vi "Trajectories2 String.vi"(5 "Trajectories":T3[](array[typedef])) -> (2 "VPL":string)   [LabVIEW 2014]
uses:
  PBFAM/Controller/MachineController/Converters/ScanSub/Trajectory.ctl
  PBFAM/Controller/MachineController/Converters/ScanSub/Path.ctl
  PBFAM/Controller/MachineController/Converters/ScanSub/Point.ctl
  PBFAM/Controller/MachineController/Converters/ScanSub/Segment.ctl
panel:
  out "Start":T1
  out "End":cluster{"X":sgl, "Y":sgl}
  out "Array":string[](array[string])
  out "Segment":T2
  out "Path0":T4
  out "Trajectory":T3
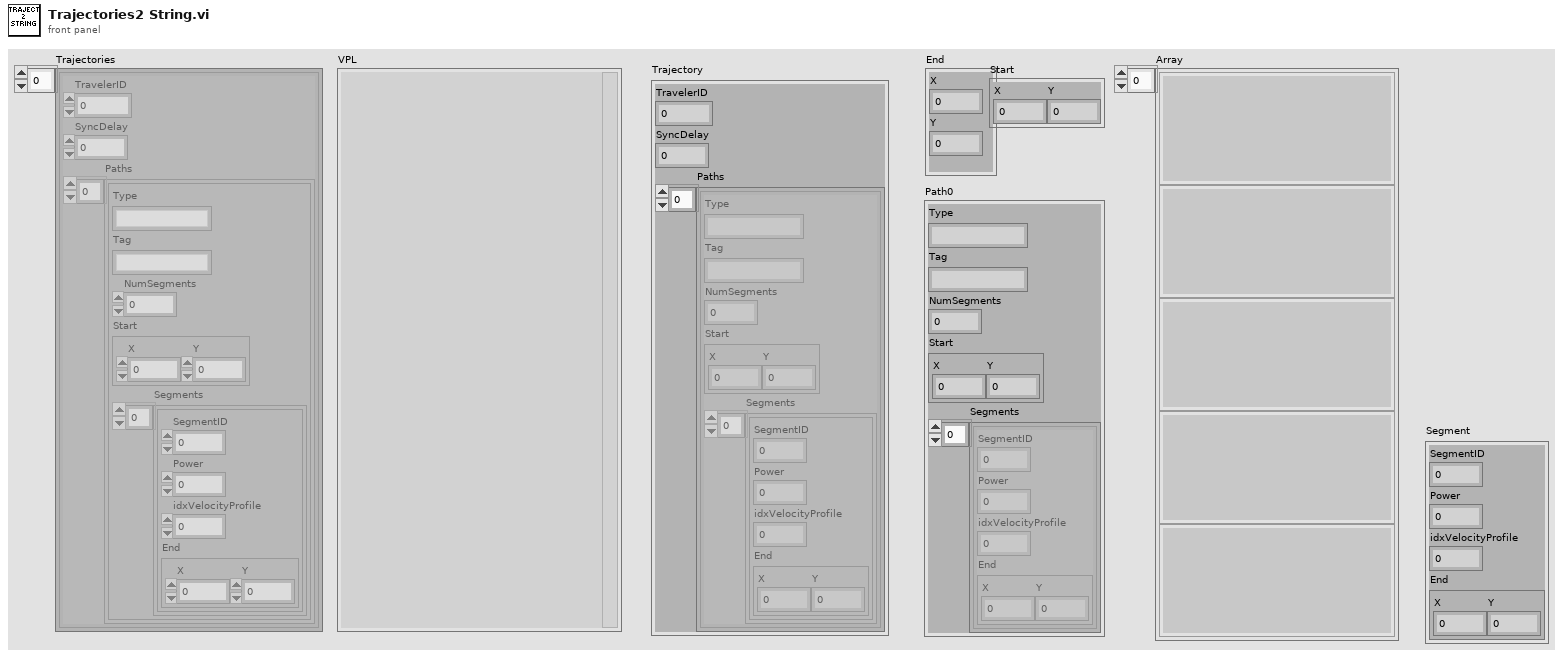
[diagram p1: front panel]
types:
  T1 = typedef "Point.ctl" = cluster{"X":dbl, "Y":dbl}
  T2 = typedef "Segment.ctl" = cluster{"SegmentID":u16, "Power":sgl, "idxVelocityProfile":u16, "End":cluster{"X":sgl, "Y":sgl}}
  T3 = typedef "Trajectory.ctl" = cluster{"TravelerID":u32, "SyncDelay":u32, "Paths":T4[]}
  T4 = typedef "Path.ctl" = cluster{"Type":string, "Tag":string, "NumSegments":u64, "Start":T1, "Segments":T2[]}
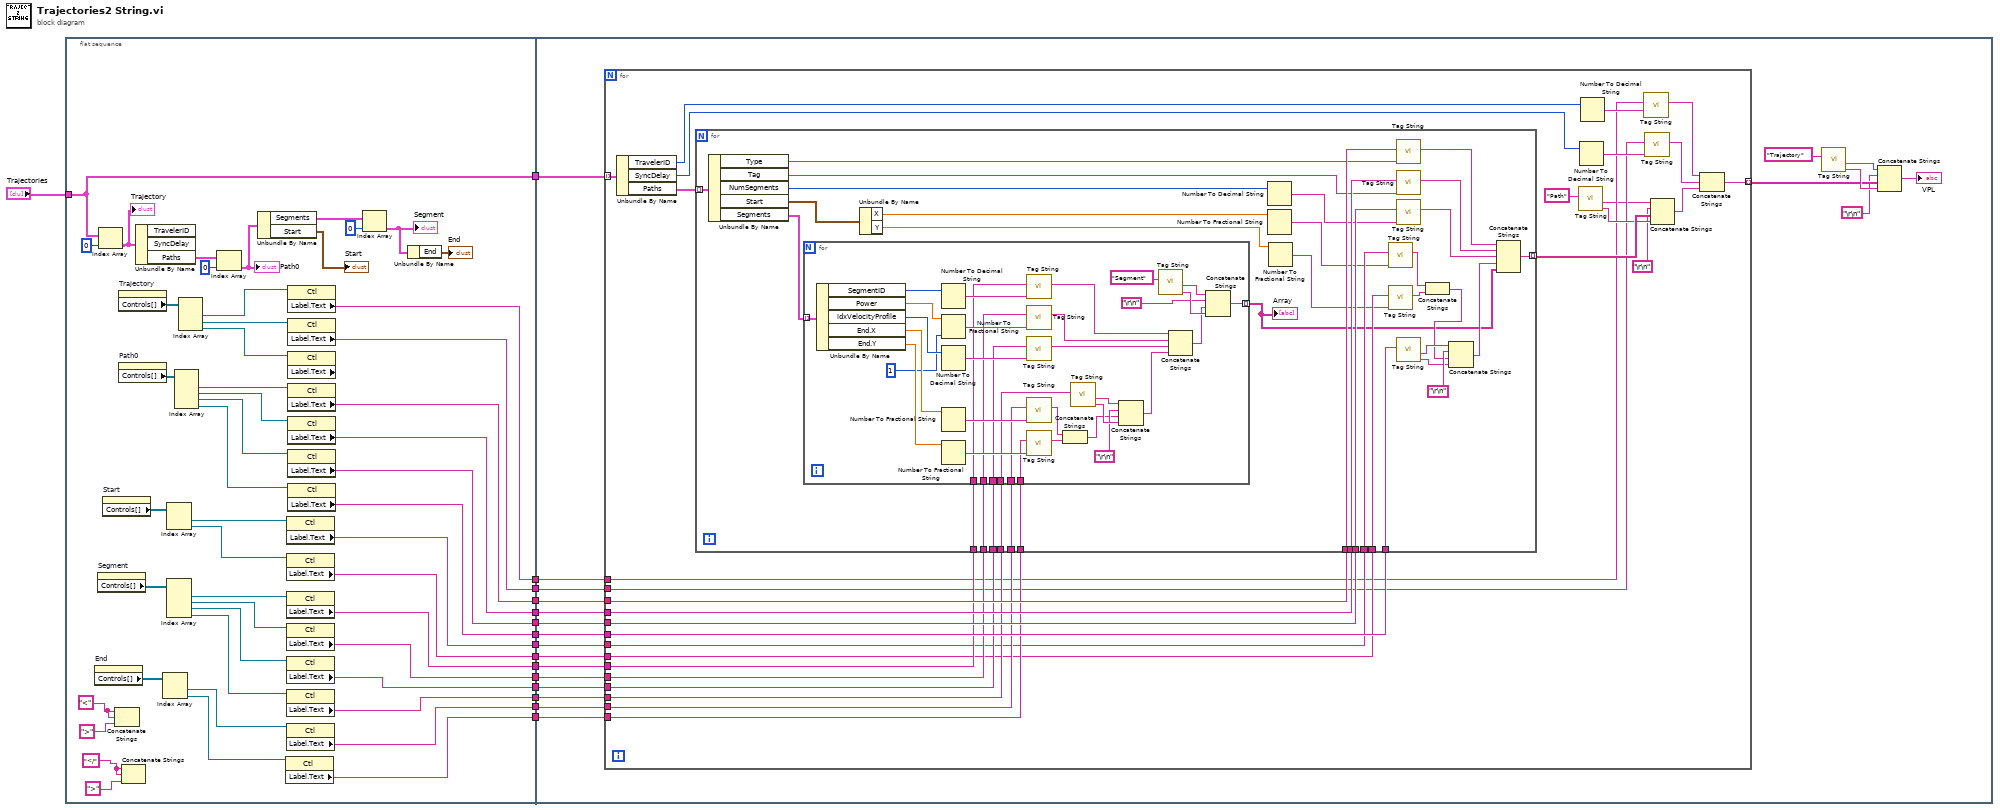
[diagram p0: block diagram]
diagram:
  n1 = flat-sequence {
    tunnel: [w53] -> w16
    tunnel: [w43] -> w15
    tunnel: [w42] -> w14
    tunnel: [w41] -> w13
    tunnel: [w40] -> w12
    tunnel: [w39] -> w11
    tunnel: [w38] -> w10
    tunnel: "Trajectories" -> [w53]
    tunnel: [w37] -> w8
    tunnel: [w36] -> w7
    tunnel: [w35] -> w6
    tunnel: [w34] -> w5
    tunnel: [w20] -> w4
    tunnel: [w19] -> w3
    tunnel: [w18] -> w2
    tunnel: [w17] -> w1
    tunnel: w16 -> [w86]
    tunnel: w15 -> [w85]
    tunnel: w14 -> [w84]
    tunnel: w13 -> [w83]
    tunnel: w12 -> [w82]
    tunnel: w11 -> [w81]
    tunnel: w10 -> [w80]
    tunnel: w8 -> [w79]
    tunnel: w7 -> [w78]
    tunnel: w6 -> [w77]
    tunnel: w5 -> [w76]
    tunnel: w4 -> [w75]
    tunnel: w3 -> [w74]
    tunnel: w2 -> [w73]
    tunnel: w1 -> [w72]
    frame #0 {
      w25 = "</" ("string")
      w26 = "<" ("string")
      n2 = property on="End" class="Clust (strict)"() -> ("Controls[]"=w31:refnum<vi>[])  [unwired: 2 in, 2 out]
      n3 = property on="Segment" class="Clust (strict)"() -> ("Controls[]"=w48:refnum<vi>[])  [unwired: 2 in, 2 out]
      n4 = Index Array(array=w53, index=0) -> (element=w52:T3)
      "Trajectory" <- w52
      n5 = property on="Start" class="Clust (strict)"() -> ("Controls[]"=w23:refnum<vi>[])  [unwired: 2 in, 2 out]
      n6 = Concatenate Strings(w26, w26, ">" ("string")) -> ()  [unwired: 1 out]
      n7 = property on="Trajectory" class="Clust (strict)"() -> ("Controls[]"=w62:refnum<vi>[])  [unwired: 2 in, 2 out]
      n8 = property on="Path0" class="Clust (strict)"() -> ("Controls[]"=w59:refnum<vi>[])  [unwired: 2 in, 2 out]
      n9 = Concatenate Strings(w25, w25, ">" ("string")) -> ()  [unwired: 1 out]
      n10 = Unbundle By Name(w52) -> ("Paths"=w61:T4[])  [unwired: 2 out]
      n11 = Index Array(array=w31) -> (element #1=w30:refnum<vi>, element #2=w29:refnum<vi>)  [unwired: 2 in]
      n12 = Index Array(array=w23) -> (element #1=w22:refnum<vi>, element #2=w21:refnum<vi>)  [unwired: 2 in]
      n13 = Index Array(array=w48) -> (element #1=w47:refnum<vi>, element #2=w46:refnum<vi>, element #3=w45:refnum<vi>, element #4=w44:refnum<vi>)  [unwired: 4 in]
      n14 = Index Array(array=w59) -> (element #1=w58:refnum<vi>, element #2=w57:refnum<vi>, element #3=w56:refnum<vi>, element #4=w55:refnum<vi>)  [unwired: 4 in]
      n15 = Index Array(array=w62) -> (element #1=w65:refnum<vi>, element #2=w64:refnum<vi>, element #3=w63:refnum<vi>)  [unwired: 3 in]
      n16 = Index Array(array=w61, index=0) -> (element=w50:T4)
      "Path0" <- w50
      n17 = Unbundle By Name(w50) -> ("Segments"=w49:T2[], "Start"=→"Start":T1)
      n18 = property class="Ctl"(reference=w29) -> ("Label.Text"=w34:string)  [unwired: 1 in, 2 out]
      n19 = property class="Ctl"(reference=w21) -> ("Label.Text"=w20:string)  [unwired: 1 in, 2 out]
      n20 = property class="Ctl"(reference=w47) -> ("Label.Text"=w39:string)  [unwired: 1 in, 2 out]
      n21 = property class="Ctl"(reference=w46) -> ("Label.Text"=w38:string)  [unwired: 1 in, 2 out]
      n22 = property class="Ctl"(reference=w45) -> ("Label.Text"=w37:string)  [unwired: 1 in, 2 out]
      n23 = property class="Ctl"(reference=w44) -> ("Label.Text"=w36:string)  [unwired: 1 in, 2 out]
      n24 = property class="Ctl"(reference=w30) -> ("Label.Text"=w35:string)  [unwired: 1 in, 2 out]
      n25 = property class="Ctl"(reference=w22) -> ("Label.Text"=w19:string)  [unwired: 1 in, 2 out]
      n26 = property class="Ctl"(reference=w65) -> ("Label.Text"=w17:string)  [unwired: 1 in, 2 out]
      n27 = property class="Ctl"(reference=w64) -> ("Label.Text"=w18:string)  [unwired: 1 in, 2 out]
      n28 = property class="Ctl" props=["Label", "Text"](reference=w63) -> ()  [unwired: 1 in, 3 out]
      n29 = property class="Ctl"(reference=w58) -> ("Label.Text"=w43:string)  [unwired: 1 in, 2 out]
      n30 = property class="Ctl"(reference=w57) -> ("Label.Text"=w42:string)  [unwired: 1 in, 2 out]
      n31 = property class="Ctl"(reference=w56) -> ("Label.Text"=w41:string)  [unwired: 1 in, 2 out]
      n32 = property class="Ctl"(reference=w55) -> ("Label.Text"=w40:string)  [unwired: 1 in, 2 out]
      n33 = Index Array(array=w49, index=0) -> (element=w33:T2)
      "Segment" <- w33
      n34 = Unbundle By Name(w33) -> ("End"=→"End":cluster{"X":sgl, "Y":sgl})
    }
    frame #1 {
      n35 = for {
        tunnel: w86 -> [w115] mode=indexing
        tunnel: w85 -> [w114]
        tunnel: w84 -> [w113]
        tunnel: w83 -> [w112]
        tunnel: w82 -> [w111]
        tunnel: w81 -> [w109]
        tunnel: w80 -> [w108]
        tunnel: w79 -> [w107]
        tunnel: w78 -> [w106]
        tunnel: w77 -> [w105]
        tunnel: w76 -> [w104]
        tunnel: w75 -> [w103]
        tunnel: w74 -> [w102]
        tunnel: w73 -> [w90]
        tunnel: w72 -> [w89]
        tunnel: [w91] -> w69 mode=indexing
        n36 = Unbundle By Name(w115) -> ("TravelerID"=w100:u32, "SyncDelay"=w101:u32, "Paths"=w110:T4[])
        n37 = for {
          tunnel: w114 -> [w150]
          tunnel: w113 -> [w149]
          tunnel: w112 -> [w148]
          tunnel: w111 -> [w128]
          tunnel: [w144] -> w96 mode=indexing
          tunnel: w110 -> [w143] mode=indexing
          tunnel: w109 -> [w134]
          tunnel: w108 -> [w133]
          tunnel: w107 -> [w132]
          tunnel: w106 -> [w131]
          tunnel: w105 -> [w130]
          tunnel: w104 -> [w129]
          tunnel: w103 -> [w126]
          tunnel: w102 -> [w127]
          n38 = Unbundle By Name(w143) -> ("Type"=w142:string, "Tag"=w141:string, "NumSegments"=w139:u64, "Start"=w138:T1, "Segments"=w135:T2[])
          n39 = for {
            tunnel: w135 -> [w184] mode=indexing
            tunnel: w134 -> [w173]
            tunnel: w133 -> [w172]
            tunnel: w132 -> [w171]
            tunnel: w131 -> [w168]
            tunnel: w130 -> [w170]
            tunnel: w129 -> [w169]
            tunnel: [w157] -> w116 mode=indexing
            n40 = Unbundle By Name(w184) -> ("SegmentID"=w183:u16, "Power"=w182:sgl, "idxVelocityProfile"=w181:u16, "End.X"=w175:sgl, "End.Y"=w174:sgl)
            n41 = Number To Decimal String(number=w183) -> (decimal integer string=w180:string)  [unwired: 1 in]
            n42 = Number To Fractional String(number=w182, precision (6)=i16 1) -> (F-format string=w179:string)  [unwired: 2 in]
            n43 = Number To Decimal String(number=w181) -> (decimal integer string=w178:string)  [unwired: 1 in]
            n44 = Number To Fractional String(number=w175) -> (F-format string=w177:string)  [unwired: 3 in]
            n45 = Number To Fractional String(number=w174) -> (F-format string=w176:string)  [unwired: 3 in]
            n46 = call "Tag String.vi"("String In"=w180, "String name"=w173) -> ("Start Tagged String Out"=w167:string)  [unwired: 3 in, 2 out]
            n47 = call "Tag String.vi"("String In"=w179, "String name"=w172) -> ("Start Tagged String Out"=w166:string)  [unwired: 3 in, 2 out]
            n48 = call "Tag String.vi"("String In"=w178, "String name"=w171) -> ("Start Tagged String Out"=w165:string)  [unwired: 3 in, 2 out]
            n49 = call "Tag String.vi"("String In"=w177, "String name"=w170) -> ("Start Tagged String Out"=w164:string)  [unwired: 3 in, 2 out]
            n50 = call "Tag String.vi"("String In"=w176, "String name"=w169) -> ("Start Tagged String Out"=w163:string)  [unwired: 3 in, 2 out]
            n51 = Concatenate Strings(w164, w163) -> (w153:string)
            n52 = call "Tag String.vi"("String name"=w168) -> ("Stop"=w156:string, "Start"=w155:string)  [unwired: 4 in, 1 out]
            n53 = Concatenate Strings(w155, "\r\n", w153, w156) -> (w152:string)
            n54 = call "Tag String.vi"("String name"="Segment") -> ("Stop"=w161:string, "Start"=w160:string)  [unwired: 4 in, 1 out]
            n55 = Concatenate Strings(w167, w166, w165, w152) -> (w158:string)
            n56 = Concatenate Strings(w160, "\r\n", w158, w161) -> (w157:string)
          }
          "Array" <- w116
          n57 = Unbundle By Name(w138) -> ("X"=w137:dbl, "Y"=w136:dbl)
          n58 = Number To Decimal String(number=w139) -> (decimal integer string=w140:string)  [unwired: 1 in]
          n59 = Number To Fractional String(number=w137) -> (F-format string=w124:string)  [unwired: 3 in]
          n60 = Number To Fractional String(number=w136) -> (F-format string=w125:string)  [unwired: 3 in]
          n61 = call "Tag String.vi"("String In"=w124, "String name"=w127) -> ("Start Tagged String Out"=w122:string)  [unwired: 3 in, 2 out]
          n62 = call "Tag String.vi"("String In"=w125, "String name"=w126) -> ("Start Tagged String Out"=w123:string)  [unwired: 3 in, 2 out]
          n63 = call "Tag String.vi"("String In"=w142, "String name"=w150) -> ("Start Tagged String Out"=w147:string)  [unwired: 3 in, 2 out]
          n64 = call "Tag String.vi"("String In"=w141, "String name"=w149) -> ("Start Tagged String Out"=w146:string)  [unwired: 3 in, 2 out]
          n65 = call "Tag String.vi"("String In"=w140, "String name"=w148) -> ("Start Tagged String Out"=w145:string)  [unwired: 3 in, 2 out]
          n66 = call "Tag String.vi"("String name"=w128) -> ("Stop"=w117:string, "Start"=w121:string)  [unwired: 4 in, 1 out]
          n67 = Concatenate Strings(w122, w123) -> (w119:string)
          n68 = Concatenate Strings(w121, "\r\n", w119, w117) -> (w118:string)
          n69 = Concatenate Strings(w147, w146, w145, w118, w116) -> (w144:string)
        }
        n70 = call "Tag String.vi"("String name"="Path") -> ("Stop"=w95:string, "Start"=w88:string)  [unwired: 4 in, 1 out]
        n71 = Number To Decimal String(number=w101) -> (decimal integer string=w98:string)  [unwired: 1 in]
        n72 = Number To Decimal String(number=w100) -> (decimal integer string=w99:string)  [unwired: 1 in]
        n73 = call "Tag String.vi"("String In"=w99, "String name"=w89) -> ("Start Tagged String Out"=w92:string)  [unwired: 3 in, 2 out]
        n74 = call "Tag String.vi"("String In"=w98, "String name"=w90) -> ("Start Tagged String Out"=w93:string)  [unwired: 3 in, 2 out]
        n75 = Concatenate Strings(w88, "\r\n", w96, w95) -> (w94:string)
        n76 = Concatenate Strings(w92, w93, w94) -> (w91:string)
      }
      n77 = call "Tag String.vi"("String name"="Trajectory") -> ("Stop"=w70:string, "Start"=w68:string)  [unwired: 4 in, 1 out]
      n78 = Concatenate Strings(w68, "\r\n", w69, w70) -> (→"VPL":string)
    }
  }
